vi "FixGotoStatements.vi"(0 "URAPI LInes":string[](array[string]), 1 "Tiny Lines":string[](array[string])) -> (2 "Bytes to EOL":i32[](array[numeric]), 3 "SubsString":string, 4 "Tiny Fixed":string[](array[string]))   [LabVIEW 2012]
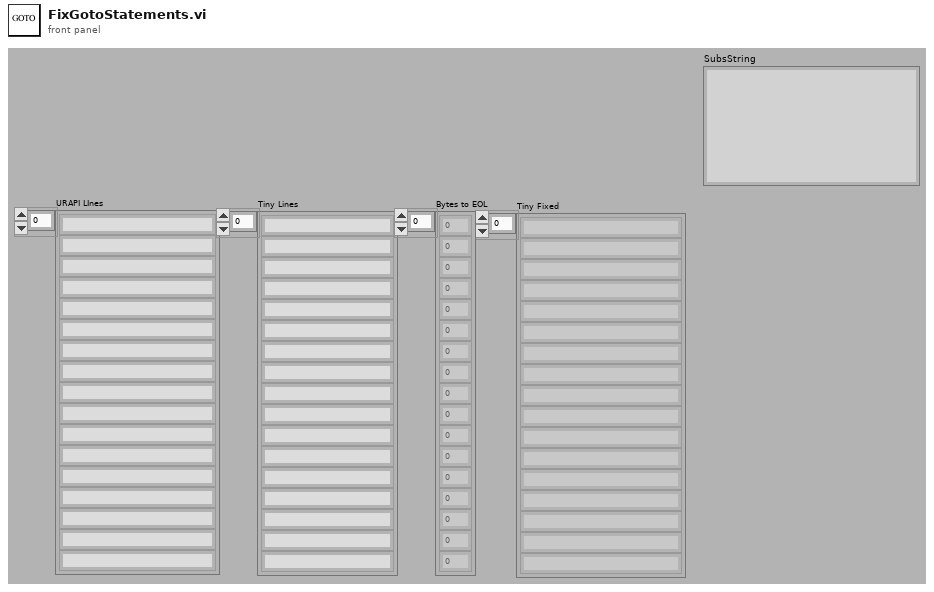
[diagram p1: front panel]
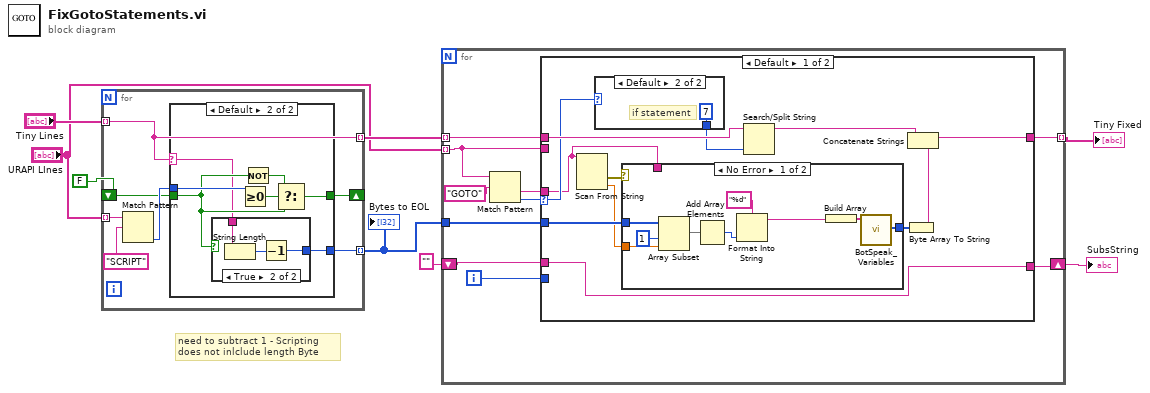
[diagram p0: block diagram]
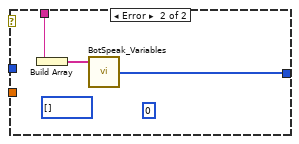
[diagram p2: hidden frame]
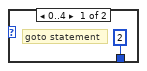
[diagram p3: hidden frame]
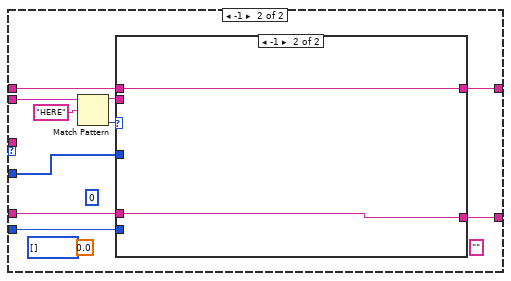
[diagram p4: hidden frame]
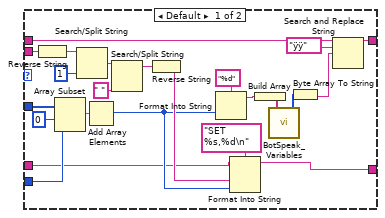
[diagram p5: hidden frame]
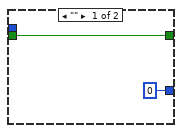
[diagram p6: hidden frame]
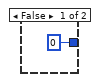
[diagram p7: hidden frame]
diagram:
  # "need to subtract 1 - Scripting \ndoes not inlclude length Byte"
  n1 = for {
    tunnel: [w9] -> w6 mode=indexing
    tunnel: [w15] -> w7 mode=indexing
    tunnel: "Tiny Lines" -> [w9] mode=indexing
    shift-right: [w12] -> _
    shift-left: FALSE -> [w11]
    tunnel: "URAPI LInes" -> [w10] mode=indexing
    n2 = Match Pattern(string=w10, regular expression="SCRIPT") -> (offset past match=w13:i32)  [unwired: 1 in, 3 out]
    n3 = case shown="Default" w9 {
      selector: w9 -> [_ w18]
      tunnel: [0 w24] -> w15
      tunnel: w13 -> [_ w22]
      tunnel: [w17 w21] -> w12
      tunnel: w11 -> [w17 w20]
      frame "" {
      }
      frame Default {
        n4 = case shown="True" w20 {
          tunnel: [0 w26] -> w24
          tunnel: w18 -> [_ w27]
          frame False {
          }
          frame True {
            n5 = String Length(string=w27) -> (length=w28:i32)
            n6 = Decrement(x=w28) -> (x-1=w26:i32)
          }
        }
        n7 = Greater Or Equal To 0?(x=w22) -> (x >= 0?=w23:bool)
        n8 = Not(x=w20) -> (.not. x?=w19:bool)
        n9 = Select(t=w19, s=w23, f=w20) -> (s? t:f=w21:bool)
      }
    }
  }
  "Bytes to EOL" <- w7
  n10 = for {
    tunnel: w6 -> [w36] mode=indexing
    tunnel: [w33] -> w1 mode=indexing
    tunnel: w7 -> [w34]
    tunnel: "URAPI LInes" -> [w31] mode=indexing
    shift-right: [w30] -> w2
    shift-left: "" -> [w29]
    i -> [w32]
    n11 = Match Pattern(string=w31, regular expression="GOTO") -> (after substring=w35:string, offset past match=w37:i32)  [unwired: 1 in, 2 out]
    n12 = case shown="Default" w37 {
      selector: w37 -> [w44 _]
      tunnel: [w49 w72] -> w33
      tunnel: w36 -> [w48 w71]
      tunnel: w35 -> [w41 _]
      tunnel: w34 -> [w50 w70]
      tunnel: w31 -> [_ w69]
      tunnel: w32 -> [_ w65]
      tunnel: [w40 w68] -> w30
      tunnel: w29 -> [w40 w67]
      frame Default {
        n13 = Scan From String(input string=w41) -> (error out=w42:errorcluster, output 1=w39:dbl)  [unwired: 4 in, 2 out]
        n14 = case shown="Default" w44 {
          tunnel: [2 ("offset (0)") 7 ("offset (0)")] -> w43
          frame 0..4 {
            # "goto statement"
          }
          frame Default {
            # "if statement"
          }
        }
        n15 = case shown="No Error" w42 {
          tunnel: w50 -> [w59 _]
          tunnel: w39 -> [w58 _]
          tunnel: [w54 w60] -> w45
          tunnel: w41 -> [_ w62]
          frame No Error {
            n16 = Array Subset(array=w59, index=1, length=w58) -> (w52:i32[])
            n17 = Add Array Elements(numeric array=w52) -> (sum=w51:i32)
            n18 = Format Into String(format string="%d", w51) -> (resulting string=w53:string)  [unwired: 2 in, 1 out]
            n19 = Build Array(w53) -> (w55:string[])
            n20 = call <userlib>:"BotSpeak_Variables.vi"("Variables"=w55) -> ("Binary out"=w54:u8[])  [unwired: 2 in]
          }
          frame Error {
            (unwired) 0
            (unwired) i32[] []
            n21 = Build Array(w62) -> (w61:string[])
            n22 = call <userlib>:"BotSpeak_Variables.vi"("Variables"=w61) -> ("Binary out"=w60:u8[])  [unwired: 2 in]
          }
        }
        n23 = Search/Split String(string=w48, offset (0)=w43) -> (substring before match=w47:string)  [unwired: 1 in, 2 out]
        n24 = Byte Array To String(unsigned byte array=w45) -> (string=w46:string)
        n25 = Concatenate Strings(w47, w46) -> (w49:string)
      }
      frame -1 {
        (unwired) 0.0
        (unwired) 0
        (unwired) i32[] []
        (unwired) ""
        n26 = Match Pattern(string=w69, regular expression="HERE") -> (before substring=w66:string, offset past match=w73:i32)  [unwired: 1 in, 2 out]
        n27 = case shown="-1" w73 {
          tunnel: [w96 w99] -> w72
          tunnel: w71 -> [w97 w99]
          tunnel: w70 -> [w89 _]
          tunnel: w66 -> [w87 _]
          tunnel: w65 -> [w80 _]
          tunnel: [w78 w98] -> w68
          tunnel: w67 -> [w75 w98]
          frame Default {
            n28 = Reverse String(1:w87) -> (0:w86:string)
            n29 = Array Subset(array=w89, index=0, length=w80) -> (w91:i32[])
            n30 = Search/Split String(string=w86, offset (0)=1) -> (match + rest of string=w84:string)  [unwired: 1 in, 2 out]
            n31 = Add Array Elements(numeric array=w91) -> (sum=w76:i32)
            n32 = Search/Split String(string=w84, search string/char (-)=" ") -> (substring before match=w81:string)  [unwired: 1 in, 2 out]
            n33 = Reverse String(1:w81) -> (0:w77:string)
            n34 = Format Into String(format string="%d", w76) -> (resulting string=w92:string)  [unwired: 2 in, 1 out]
            n35 = Format Into String(format string="SET %s,%d\n", initial string=w75, w77, w76) -> (resulting string=w78:string)  [unwired: 1 in, 1 out]
            n36 = Build Array(w92) -> (w93:string[])
            n37 = call <userlib>:"BotSpeak_Variables.vi"("Variables"=w93) -> ("Binary out"=w94:u8[])  [unwired: 2 in]
            n38 = Byte Array To String(unsigned byte array=w94) -> (string=w88:string)
            n39 = Search and Replace String(input string=w97, search string="ÿÿ", replace string=w88) -> (result string=w96:string)  [unwired: 5 in, 3 out]
          }
          frame -1 {
          }
        }
      }
    }
  }
  "Tiny Fixed" <- w1
  "SubsString" <- w2
